vi "IBM4_Find_COM_port.vi"() -> (0 "error out":errorcluster, 3 "COM resource out":refnum<visa-resource-name>)   [LabVIEW 2023, in "IBM4.lvlib"]
doc: "This VI searches for the first available IBM4 and then opens it.\nIf the code returns and error, then there are now IBM4s available with the correct UCC source code."
uses:
  <instrlib>/IBM4/IBM4.lvlib
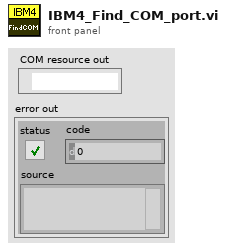
[diagram p1: front panel]
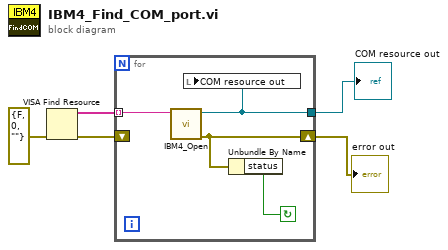
[diagram p0: block diagram]
diagram:
  n1 = VISA Find Resource(8:errorcluster {"status"=FALSE, "code"=0, "source"=""} ("error in (no error)")) -> (0:w3:errorcluster, 3:w4:string[])  [unwired: 2 in, 1 out]
  n2 = for {
    tunnel: w4 -> [w9] mode=indexing
    shift-right: [w8] -> w2
    shift-left: w3 -> [_]
    tunnel: [w6] -> w1
    stop <- w7 continue-if-true
    n3 = call <instrlib>:"IBM4_Open.vi"("COM Port"=w9) -> ("error out"=w8:errorcluster, "COM resource out"=w6:refnum<visa-resource-name>)  [unwired: 8 in, 1 out]
    n4 = local write "COM resource out"(w6) -> ()
    n5 = Unbundle By Name(w8) -> ("status"=w7:bool)
  }
  "error out" <- w2
  "COM resource out" <- w1
